vi "Signal Analyzer.vi"(4 "Period [ms]":i64=40, 5 "Current [pA]":refnum<vi>, 6 "Controllers":T2, 7 "Resistance [MOhm]":refnum<vi>, 8 "error in (no error)":errorcluster, 9 "Amplitude [mV]":refnum<vi>, 10 "Gain":refnum<vi>, 11 "Test Signal":refnum<vi>) -> (0 "error out":errorcluster)   [LabVIEW 2012, in "Signal Analysis.lvlib"]
uses:
  Signal Analysis.lvlib
  <vilib>/Analysis/baseanly.llb/Mean (DBL).vi
  <vilib>/measure/macond.llb/IIR Filter for 1 Chan.vi
  <vilib>/Analysis/NI_AALBase.lvlib
  <vilib>/measure/NI_MAPro.lvlib
panel:
  out "Exit":bool
  out "Amplitude [V]":dbl
  out "Gain":dbl
  out "Test Signal":waveform(dbl)
  out "Filter Specs":T1
  in  "Current":dbl
  in  "Resistance":dbl
  out "Filter":bool
  out "On/Off":bool
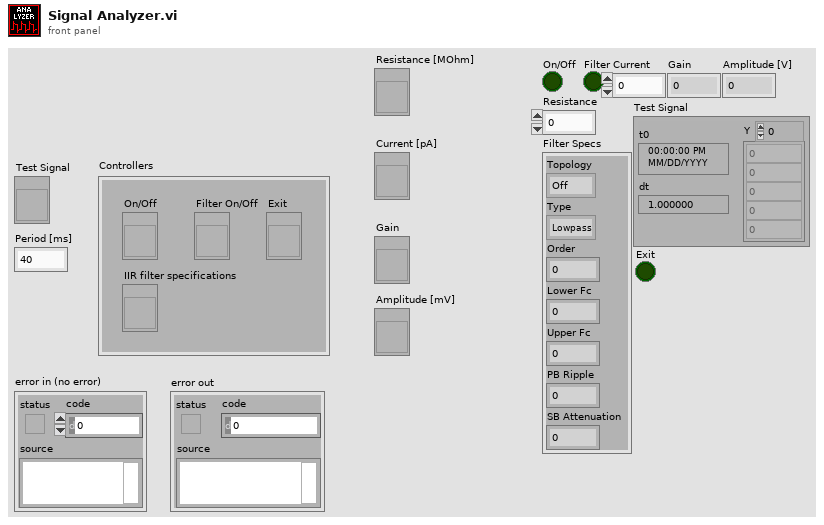
[diagram p1: front panel]
types:
  T1 = cluster{"Topology":enum16{"Off", "Butterworth", "Chebyshev", "Inverse Chebyshev", "Elliptic", "Bessel"}, "Type":enum16{"Lowpass", "Highpass", "Bandpass", "Bandstop"}, "Order":i32, "Lower Fc":dbl, "Upper Fc":dbl, "PB Ripple":dbl, "SB Attenuation":dbl}
  T2 = cluster{"On/Off":refnum<vi>, "Filter On/Off":refnum<vi>, "Exit":refnum<vi>, "IIR filter specifications":refnum<vi>}
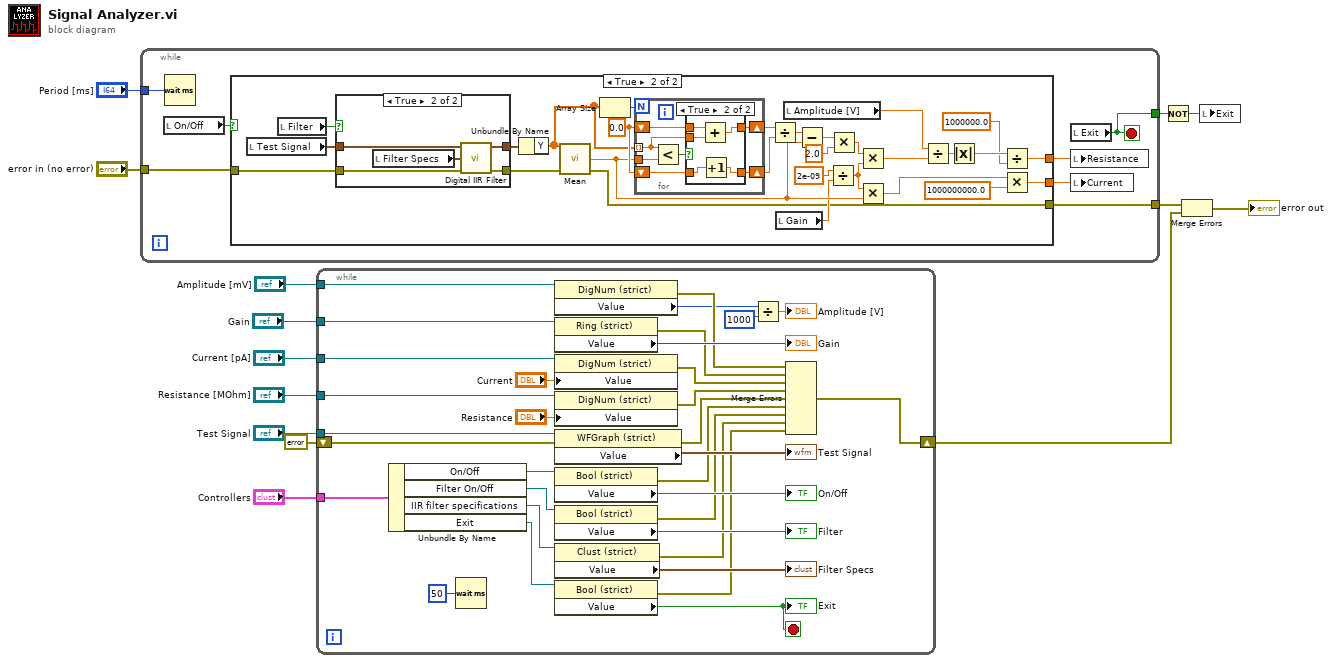
[diagram p0: block diagram]
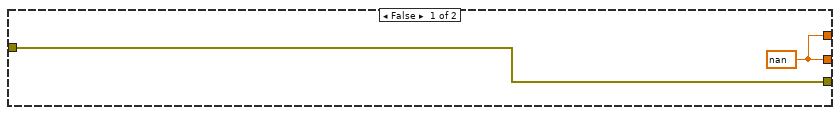
[diagram p2: hidden frame]
diagram:
  n1 = while {
    tunnel: [w18] -> w13
    tunnel: [w17] -> w6
    tunnel: "error in (no error)" -> [w16]
    tunnel: "Period [ms]" -> [w15]
    stop <- w18 stop-if-true
    n2 = local read "On/Off"() -> (w19:bool)
    n3 = Wait (ms)(milliseconds to wait=w15) -> ()  [unwired: 1 out]
    n4 = case shown="True" w19 {
      tunnel: [w22 w24] -> w17
      tunnel: w16 -> [w22 w50]
      tunnel: [w23 w49] -> w21
      tunnel: [w23 w48] -> w20
      frame False {
        w23 = nan
      }
      frame True {
        w44 = 0.0
        n5 = local read "Test Signal"() -> (w27:waveform(dbl))
        n6 = local read "Filter"() -> (w28:bool)
        n7 = case shown="True" w28 {
          tunnel: w50 -> [w51 w57]
          tunnel: w27 -> [w52 w56]
          tunnel: [w52 w55] -> w41
          tunnel: [w51 w54] -> w24
          frame False {
          }
          frame True {
            n8 = local read "Filter Specs"() -> (w53:T1)
            n9 = call-poly <vilib>:"Digital IIR Filter.vi"("IIR filter specifications"=w53, "error in (no error)"=w57, "signal in"=w56) -> ("error out"=w54:errorcluster, "signal out"=w55:waveform(dbl))  [unwired: 6 in, 1 out]
          }
        }
        n10 = Unbundle By Name(w41) -> ("Y"=w29:dbl[])
        n11 = call-poly <vilib>:"Mean.vi"("X"=w29) -> ("mean"=w40:dbl)  [unwired: 1 out]
        n12 = Array Size(array=w29) -> (size(s)=w46:i32)
        n13 = for {
          N: w46 -> [_]
          tunnel: w29 -> [w60] mode=indexing
          tunnel: w40 -> [w64]
          shift-right: [w61] -> w45
          shift-left: w44 -> [w62]
          shift-right: [w58] -> w43
          shift-left: w44 -> [w59]
          n14 = Less?(x=w60, y=w64) -> (x < y?=w63:bool)
          n15 = case shown="True" w63 {
            tunnel: w62 -> [w66 w71]
            tunnel: [w66 w70] -> w61
            tunnel: w60 -> [_ w67]
            tunnel: w59 -> [w65 w69]
            tunnel: [w65 w68] -> w58
            frame False {
            }
            frame True {
              n16 = Add(x=w71, y=w67) -> (x+y=w70:dbl)
              n17 = Increment(x=w69) -> (x+1=w68:dbl)
            }
          }
        }
        n18 = Divide(x=w45, y=w43) -> (x/y=w42:dbl)
        n19 = local read "Gain"() -> (w26:dbl)
        n20 = local read "Amplitude [V]"() -> (w25:dbl)
        n21 = Subtract(x=w42, y=w40) -> (x-y=w36:dbl)
        n22 = Divide(x=2e-09 ("y"), y=w26) -> (x/y=w30:dbl)
        n23 = Multiply(x=w36, y=2.0) -> (x*y=w38:dbl)
        n24 = Multiply(x=w38, y=w30) -> (x*y=w39:dbl)
        n25 = Multiply(x=w30, y=w40) -> (x*y=w33:dbl)
        n26 = Divide(x=w25, y=w39) -> (x/y=w47:dbl)
        n27 = Absolute Value(x=w47) -> (abs(x)=w35:dbl)
        n28 = Divide(x=w35, y=1000000.0) -> (x/y=w49:dbl)
        n29 = Multiply(x=w33, y=1000000000.0) -> (x*y=w48:dbl)
      }
    }
    n30 = local read "Exit"() -> (w18:bool)
    n31 = local write "Resistance"(w21) -> ()
    n32 = local write "Current"(w20) -> ()
  }
  n33 = while {
    tunnel: "Test Signal" -> [w97]
    tunnel: "Controllers" -> [w95]
    tunnel: "Resistance [MOhm]" -> [w82]
    tunnel: "Current [pA]" -> [w92]
    shift-right: [w91] -> w7
    shift-left: errorcluster {"status"=FALSE, "code"=0, "source"=""} ("error IO") -> [w75]
    tunnel: "Gain" -> [w80]
    tunnel: "Amplitude [mV]" -> [w79]
    stop <- w104 stop-if-true
    n34 = Unbundle By Name(w95) -> ("On/Off"=w103:refnum<vi>, "Filter On/Off"=w94:refnum<vi>, "IIR filter specifications"=w100:refnum<vi>, "Exit"=w93:refnum<vi>)
    n35 = Wait (ms)(milliseconds to wait=u32 50) -> ()  [unwired: 1 out]
    n36 = property class="DigNum (strict)"(reference=w79) -> (error out=w76:errorcluster, "Value"=w74:i32)  [unwired: 1 in, 1 out]
    n37 = property class="Ring (strict)"(reference=w80) -> (error out=w77:errorcluster, "Value"=→"Gain":u16)  [unwired: 1 in, 1 out]
    n38 = property class="DigNum (strict)"(reference=w92, "Value"="Current") -> (error out=w90:errorcluster)  [unwired: 1 in, 1 out]
    n39 = property class="DigNum (strict)"(reference=w82, "Value"="Resistance") -> (error out=w89:errorcluster)  [unwired: 1 in, 1 out]
    n40 = property class="WFGraph (strict)"(reference=w97, error in=w75) -> (error out=w88:errorcluster, "Value"=→"Test Signal":waveform(dbl))  [unwired: 1 out]
    n41 = property class="Bool (strict)"(reference=w103) -> (error out=w87:errorcluster, "Value"=→"On/Off":bool)  [unwired: 1 in, 1 out]
    n42 = property class="Bool (strict)"(reference=w94) -> (error out=w86:errorcluster, "Value"=→"Filter":bool)  [unwired: 1 in, 1 out]
    n43 = property class="Clust (strict)"(reference=w100) -> (error out=w85:errorcluster, "Value"=→"Filter Specs":T1)  [unwired: 1 in, 1 out]
    n44 = property class="Bool (strict)"(reference=w93) -> (error out=w84:errorcluster, "Value"=w104:bool)  [unwired: 1 in, 1 out]
    "Exit" <- w104
    n45 = Divide(x=w74, y=1000) -> (x/y=→"Amplitude [V]":dbl)
    n46 = Merge Errors(w76, w77, w90, w89, w88, w87, w86, w85, w84) -> (w91:errorcluster)
  }
  n47 = Not(x=w13) -> (.not. x?=w12:bool)
  n48 = Merge Errors(w6, w7) -> (→"error out":errorcluster)
  n49 = local write "Exit"(w12) -> ()
